vi "Flat_Sequence_Dependiente.vi"() -> ()   [LabVIEW 2016]
panel:
  out "x+y 2":dbl
  out "Triangle 2":dynamicdata(graph) caption="Triangle"
  out "Sine 2":dynamicdata(graph) caption="Sine"
  out "x+y":dbl
  out "Triangle":dynamicdata(graph)
  out "Sine":dynamicdata(graph)
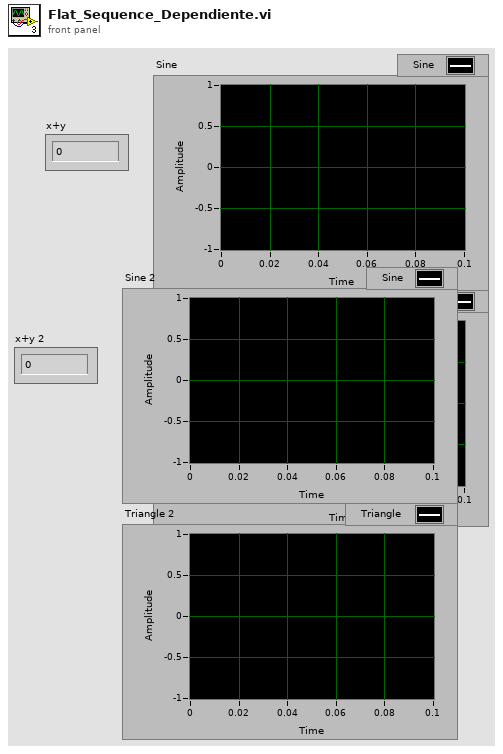
[diagram p1: front panel]
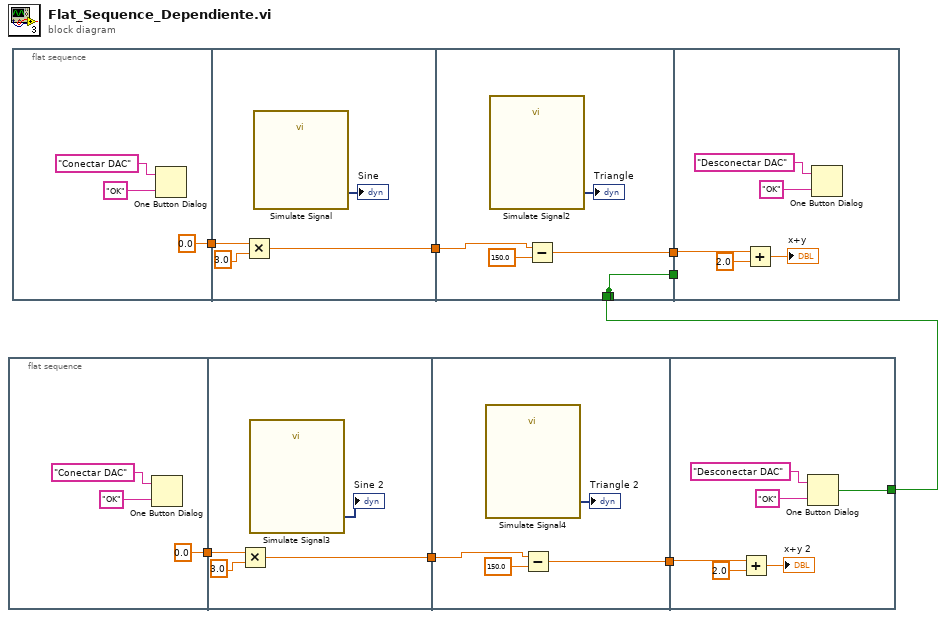
[diagram p0: block diagram]
diagram:
  n1 = flat-sequence {
    tunnel: [0.0] -> w5
    tunnel: w5 -> [w13]
    tunnel: [w12] -> w4
    tunnel: w4 -> [w17]
    tunnel: [w16] -> w3
    tunnel: w3 -> [w23]
    tunnel: [w20] -> w2
    frame #0 {
      n2 = One Button Dialog(message="Conectar DAC", button name ("OK")="OK") -> ()  [unwired: 1 out]
    }
    frame #1 {
      n3 = Multiply(x=w13, y=3.0) -> (x*y=w12:dbl)
      n4 = call "Simulate Signal3"() -> ("Sine"=→"Sine 2":dynamicdata)  [unwired: 14 in, 1 out]
    }
    frame #2 {
      n5 = call "Simulate Signal4"() -> ("Triangle"=→"Triangle 2":dynamicdata)  [unwired: 14 in, 1 out]
      n6 = Subtract(x=w17, y=150.0) -> (x-y=w16:dbl)
    }
    frame #3 {
      n7 = Add(x=w23, y=2.0) -> (x+y=→"x+y 2":dbl)
      n8 = One Button Dialog(message="Desconectar DAC", button name ("OK")="OK") -> (true=w20:bool)
    }
  }
  n9 = flat-sequence {
    tunnel: [0.0] -> w8
    tunnel: w8 -> [w30]
    tunnel: [w29] -> w7
    tunnel: w7 -> [w35]
    tunnel: [w34] -> w6
    tunnel: [w33] -> _
    tunnel: w2 -> [w33]
    tunnel: [w33] -> w1
    tunnel: w6 -> [w40]
    tunnel: w1 -> [_]
    frame #0 {
      n10 = One Button Dialog(message="Conectar DAC", button name ("OK")="OK") -> ()  [unwired: 1 out]
    }
    frame #1 {
      n11 = Multiply(x=w30, y=3.0) -> (x*y=w29:dbl)
      n12 = call "Simulate Signal"() -> ("Sine"=→"Sine":dynamicdata)  [unwired: 14 in, 1 out]
    }
    frame #2 {
      n13 = call "Simulate Signal2"() -> ("Triangle"=→"Triangle":dynamicdata)  [unwired: 14 in, 1 out]
      n14 = Subtract(x=w35, y=150.0) -> (x-y=w34:dbl)
    }
    frame #3 {
      n15 = Add(x=w40, y=2.0) -> (x+y=→"x+y":dbl)
      n16 = One Button Dialog(message="Desconectar DAC", button name ("OK")="OK") -> ()  [unwired: 1 out]
    }
  }
